vi "Back half.vi"() -> ()   [LabVIEW 2013]
panel:
  in  "VLS Valves":bool=TRUE
  out "TI-640":dbl format="%.1f"
  out "TI-630":dbl format="%.1f"
  in  "XV-641":bool
  in  "XV-640":bool
  in  "XV-630":bool
  out "PI-641":dbl format="%.1f"
  out "TI-641":dbl format="%.1f"
  out "FI-641":dbl format="%.1f"
  out "TI-631":dbl format="%.1f"
  out "1 LO":bool
  out "1 HI":bool
  out "2 LO":bool
  out "2 HI":bool
  in  "PCV-641":dbl format="%.2f"
  out "PCV-641 PV":dbl format="%.2f"
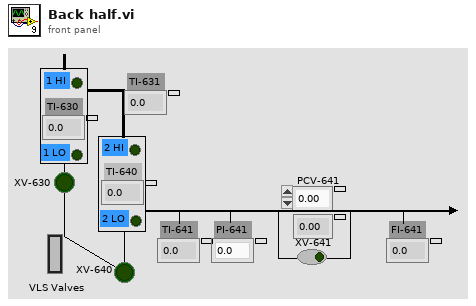
[diagram p1: front panel]
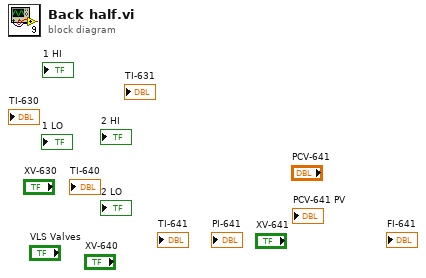
[diagram p0: block diagram]
diagram:
